vi "tb_dsp48 subtract.vi"() -> ()   [LabVIEW 2011]
uses:
  <vilib>/rvi/FXPMathLib/FxpConvert/subVIs/nifxpmath_Convert_SimConfig.ctl
  <vilib>/fxp/LVFixedPointQuantizationPolicyTypeDef.ctl
  <vilib>/fxp/LVFixedPointOverflowPolicyTypeDef.ctl
  <vilib>/rvi/FXPMathLib/FxpConvert/simVIs/DllFxpConvertTemp_sub.vi
  <vilib>/rvi/FXPMathLib/FxpInterpret/XNode/nifxpmath_Interpret.xnode
  <vilib>/rvi/FXPMathLib/FxpConvert/XNode/nifxpmath_Convert.xnode
panel:
  in  "B":fxp<+/-,16,16>
  out "A-B":fxp<+/-,48,24> format="%.6g"
  in  "A":fxp<+/-,48,24>
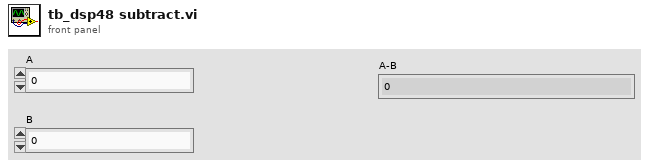
[diagram p1: front panel]
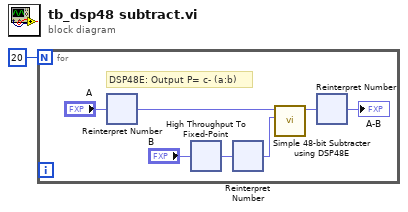
[diagram p0: block diagram]
diagram:
  n1 = for {
    N: 20 -> [_]
    # "DSP48E: Output P= c- (a:b)"
    n2 = xnode "Reinterpret Number"("x"="A") -> ("y"=w6:fxp<+/-,48,48>)
    n3 = xnode "High Throughput To Fixed-Point"("x"="B") -> ("y"=w2:fxp<+/-,48,24>)
    n4 = xnode "Reinterpret Number"("x"=w2) -> ("y"=w5:fxp<+/-,48,48>)
    n5 = call <userlib>:"Simple 48-bit Subtracter using DSP48E.vi"("A2"=w5, "A1"=w6) -> ("A1-A2"=w4:fxp<+/-,48,48>)  [unwired: 8 in, 1 out]
    n6 = xnode "Reinterpret Number"("x"=w4) -> ("y"=→"A-B":fxp<+/-,48,24>)
  }
